vi "SV Test for Measurement Settled (1 Ch) (Array) (DBL).vi"(8 "error in (no error)":errorcluster, 10 "settling configuration":T1={"target value"=inf, "tolerance"=1.0, "units"=1, "normalized time constant\n[samples]"=0.0, "mask length [samples]"=0} {"target value" format="%_4g"; "mask length [samples]" min=-1 step=1; "normalized time constant\n[samples]" format="%_4g"; "units" items=["Input units", "% of target"]; "tolerance" format="%_4g"}, 11 "data in":dbl[](array[numeric])) -> (0 "error out":errorcluster, 1 "output values":dbl[][](graph), 2 "point results":bool[](array[boolean]), 3 "settled?":bool)   [LabVIEW 2017]
doc: "Use this VI to test a settled double-precision output of an input array or waveform. Use the <B>settling configuration</B> input to configure the settling mask parameters. <B>output values</B> returns the thresholds and failures from the settling mask. Use the waveform instance of this VI to test waveform input."
uses:
  <vilib>/addons/Sound and Vibration/svt_Limit Test/SoundVib_LimitTest.lvlib
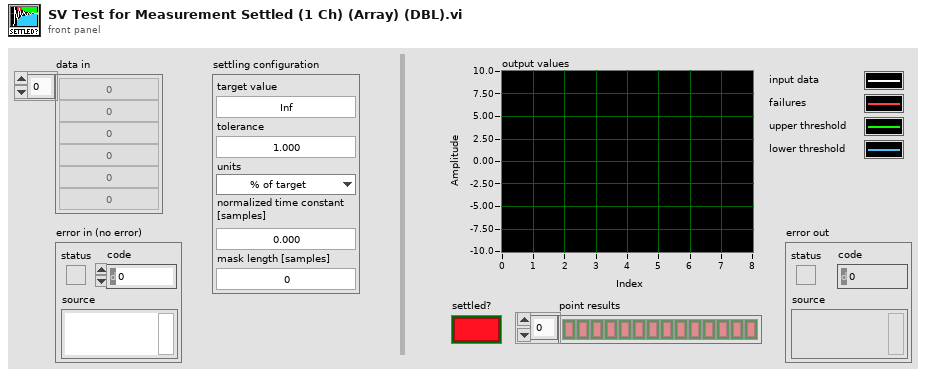
[diagram p1: front panel]
types:
  T1 = cluster{"target value":dbl, "tolerance":dbl, "units":u16, "normalized time constant\n[samples]":dbl, "mask length [samples]":i32}
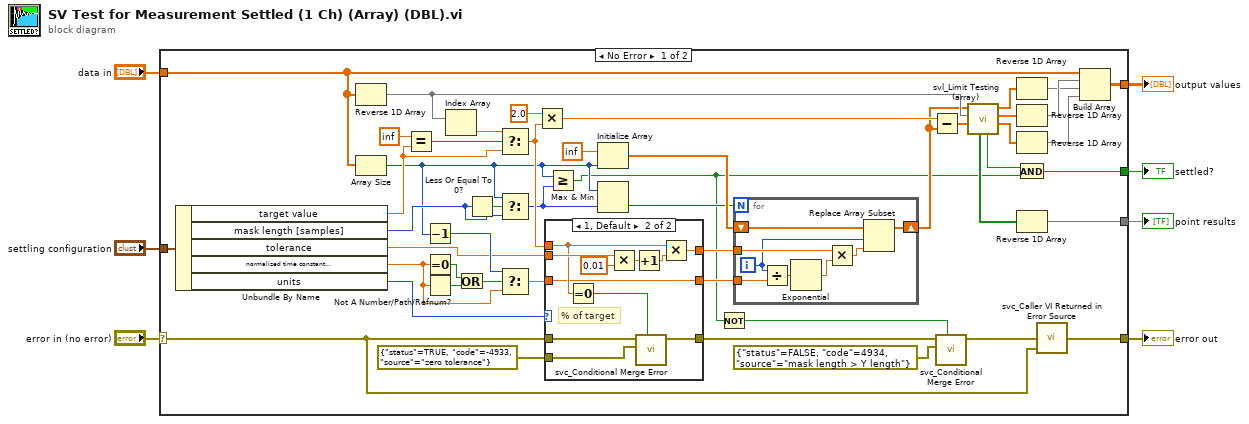
[diagram p0: block diagram]
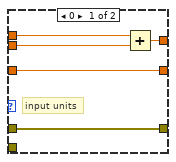
[diagram p2: hidden frame]
diagram:
  n1 = case shown="No Error" "error in (no error)" {
    selector: "error in (no error)" -> [w18 w80]
    tunnel: [w16 _] -> w7
    tunnel: [w35 _] -> w6
    tunnel: "data in" -> [w45 _]
    tunnel: [w41 _] -> w4
    tunnel: [w37 w80] -> w2
    tunnel: "settling configuration" -> [w24 _]
    frame No Error {
      n2 = Unbundle By Name(w24) -> ("target value"=w23:dbl, "mask length [samples]"=w22:i32, "tolerance"=w21:dbl, "normalized time constant\n[samples]"=w20:dbl, "units"=w19:u16)
      n3 = Reverse 1D Array(array=w45) -> (reversed array=w39:dbl[])
      n4 = Array Size(array=w45) -> (size(s)=w14:i32)
      n5 = Equal?(x=inf ("y"), y=w23) -> (x = y?=w54:bool)
      n6 = Decrement(x=w14) -> (x-1=w52:i32)
      n7 = Equal To 0?(x=w20) -> (x = 0?=w50:bool)
      n8 = Not A Number/Path/Refnum?(number/path/refnum=w20) -> (NaN/Path/Refnum?=w51:bool)
      n9 = Index Array(array=w39) -> (element=w53:dbl)  [unwired: 1 in]
      n10 = Or(x=w50, y=w51) -> (x .or. y?=w49:bool)
      n11 = Less Or Equal To 0?(x=w22) -> (x <= 0?=w34:bool)
      n12 = Select(t=w53, s=w54, f=w23) -> (s? t:f=w38:dbl)
      n13 = Select(t=w14, s=w34, f=w22) -> (s? t:f=w15:i32)
      n14 = Select(t=w52, s=w49, f=w20) -> (s? t:f=w30:dbl)
      n15 = Multiply(x=2.0 ("y"), y=w38) -> (x*y=w32:dbl)
      n16 = case shown="1, Default" w19 {
        tunnel: w38 -> [w60 w66]
        tunnel: w21 -> [w59 w71]
        tunnel: [w58 w70] -> w31
        tunnel: w30 -> [w57 w65]
        tunnel: [w57 w65] -> w29
        tunnel: [w56 w64] -> w13
        tunnel: w18 -> [w56 w63]
        tunnel: errorcluster {"status"=TRUE, "code"=-4933, "source"="zero tolerance"} ("error in") -> [_ w61]
        frame 0 {
          # "input units"
          n17 = Add(x=w60, y=w59) -> (x+y=w58:dbl)
        }
        frame 1, Default {
          # "% of target"
          n18 = Equal To 0?(x=w66) -> (x = 0?=w62:bool)
          n19 = Multiply(x=w71, y=0.01) -> (x*y=w69:dbl)
          n20 = Increment(x=w69) -> (x+1=w67:dbl)
          n21 = call <vilib>:"svc_Conditional Merge Error.vi"("merge"=w62, "new error"=w61, "error in (no error)"=w63) -> ("error out"=w64:errorcluster)  [unwired: 8 in]
          n22 = Multiply(x=w66, y=w67) -> (x*y=w70:dbl)
        }
      }
      n23 = Greater Or Equal?(x=w14, y=w15) -> (x >= y?=w11:bool)
      n24 = Initialize Array(inf ("element"), w14) -> (w27:dbl[])
      n25 = Max & Min(x=w14, y=w15) -> (min(x,y)=w25:i32)  [unwired: 1 out]
      n26 = Not(x=w11) -> (.not. x?=w10:bool)
      n27 = for {
        N: w25 -> [_]
        tunnel: w29 -> [w79]
        tunnel: w31 -> [w76]
        shift-right: [w72] -> w26
        shift-left: w27 -> [w75]
        i -> [w74]
        n28 = Divide(x=w74, y=w79) -> (x/y=w78:dbl)
        n29 = Exponential(1:w78) -> (0:w77:dbl)
        n30 = Multiply(x=w76, y=w77) -> (x*y=w73:dbl)
        n31 = Replace Array Subset(array=w75, new element=w73, index=w74) -> (w72:dbl[])
      }
      n32 = Subtract(x=w32, y=w26) -> (x-y=w40:dbl[])
      n33 = call <vilib>:"svc_Conditional Merge Error.vi"("merge"=w10, "new error"=errorcluster {"status"=FALSE, "code"=4934, "source"="mask length > Y length"} ("error in"), "error in (no error)"=w13) -> ("error out"=w9:errorcluster)  [unwired: 8 in]
      n34 = call <vilib>:"svl_Limit Testing (array).vi"("lower limit"=w40, "input array"=w39, "upper limit"=w26) -> ("dup lower limit"=w47:dbl[], "failure array"=w46:dbl[], "dup upper limit"=w48:dbl[], "test passed"=w17:bool, "test results"=w36:bool[])  [unwired: 4 in]
      n35 = Reverse 1D Array(array=w48) -> (reversed array=w43:dbl[])
      n36 = Reverse 1D Array(array=w46) -> (reversed array=w44:dbl[])
      n37 = Reverse 1D Array(array=w47) -> (reversed array=w42:dbl[])
      n38 = And(x=w17, y=w11) -> (x .and. y?=w16:bool)
      n39 = Reverse 1D Array(array=w36) -> (reversed array=w35:bool[])
      n40 = call <vilib>:"svc_Caller VI Returned in Error Source.vi"("warning input to caller"=w18, "error in (no error)"=w9) -> ("error out"=w37:errorcluster)  [unwired: 3 in]
      n41 = Build Array(w45, w44, w43, w42) -> (w41:dbl[][])
    }
    frame Error {
    }
  }
  "settled?" <- w7
  "point results" <- w6
  "output values" <- w4
  "error out" <- w2
